vi "FGV - FB.vi"(0 "System FB":bool[](array[boolean]), 1 "Supply 1 Voltage":u32, 2 "Action":T1=enum."R", 5 "Fault FB":bool[](array[boolean]), 7 "Flash FB":bool[](array[boolean]), 9 "CMD FB":bool[](array[boolean]), 11 "error in (no error)":errorcluster, 12 "Supply 2 Voltage":u32) -> (3 "Supply 1 Voltage":u32, 4 "CMD FB":bool[](array[boolean]), 6 "Fault FB":bool[](array[boolean]), 8 "Flash FB":bool[](array[boolean]), 10 "System FB":bool[](array[boolean]), 14 "Supply 2 Voltage":u32, 15 "error out":errorcluster)   [LabVIEW 2018]
uses:
  CTL/FGV - R-W.ctl
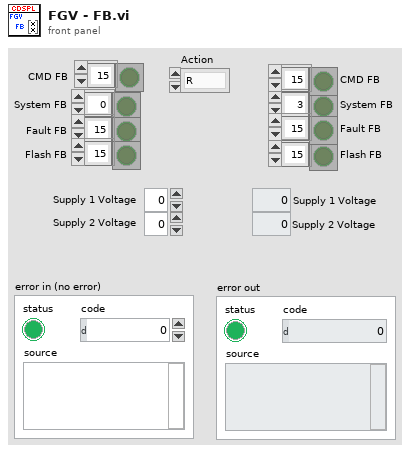
[diagram p1: front panel]
types:
  T1 = typedef "FGV - R-W.ctl" = enum16{"W", "R"}
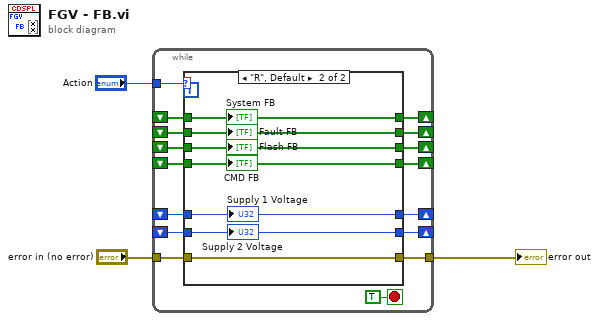
[diagram p0: block diagram]
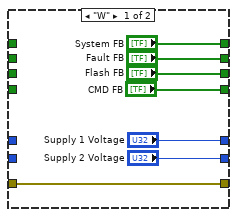
[diagram p2: hidden frame]
diagram:
  n1 = while {
    tunnel: "Action" -> [w19]
    tunnel: "error in (no error)" -> [w18]
    tunnel: [w17] -> w1
    shift-right: [w16] -> _
    shift-left: _ -> [w15]
    shift-right: [w13] -> _
    shift-left: _ -> [w12]
    shift-right: [w11] -> _
    shift-left: _ -> [w6]
    shift-right: [w9] -> _
    shift-left: _ -> [w7]
    shift-right: [w10] -> _
    shift-left: _ -> [w8]
    shift-right: [w4] -> _
    shift-left: _ -> [w5]
    stop <- TRUE stop-if-true
    n2 = case shown="\"R\", Default" w19 {
      tunnel: [w26 w33] -> w17
      tunnel: w18 -> [w26 w33]
      tunnel: ["System FB" w28] -> w16
      tunnel: w15 -> [_ w28]
      tunnel: ["Fault FB" w29] -> w13
      tunnel: w12 -> [_ w29]
      tunnel: ["Flash FB" w30] -> w11
      tunnel: ["Supply 1 Voltage" w32] -> w10
      tunnel: ["Supply 2 Voltage" w31] -> w9
      tunnel: w8 -> [_ w32]
      tunnel: w7 -> [_ w31]
      tunnel: w6 -> [_ w30]
      tunnel: w5 -> [_ w27]
      tunnel: ["CMD FB" w27] -> w4
      frame "W" {
      }
      frame "R", Default {
        "System FB" <- w28
        "Fault FB" <- w29
        "Flash FB" <- w30
        "Supply 2 Voltage" <- w31
        "Supply 1 Voltage" <- w32
        "CMD FB" <- w27
      }
    }
  }
  "error out" <- w1
